vi "Matches.vi"(8 "error in (no error)":errorcluster, 10 "Actual":variant, 11 "Constraint in":refnum<class "Constraint.lvclass">) -> (0 "error out":errorcluster, 2 "Result":bool, 3 "Constraint out":refnum<class "Constraint.lvclass">)   [LabVIEW 2019, in "Constraint.lvlib" / "Constraint.lvclass"]
doc: "Evaluates the constraint for <B>Actual</B>. Returns true if the constraint is met."
uses:
  Constraint.lvclass
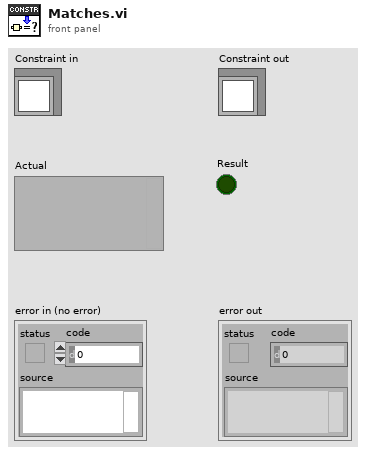
[diagram p1: front panel]
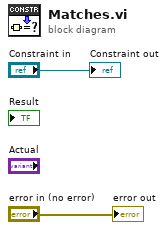
[diagram p0: block diagram]
diagram:
  "error out" <- "error in (no error)"
  "Constraint out" <- "Constraint in"
